vi "Untitled 5.vi"() -> ()   [LabVIEW 2023]
panel:
  in  "index":i8
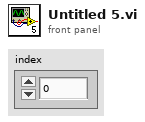
[diagram p1: front panel]
types:
  T1 = enum16{"plate1", "plate2", "plate3", "rinse", "seat"}
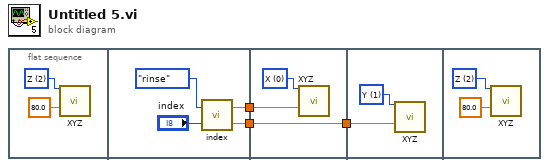
[diagram p0: block diagram]
diagram:
  n1 = flat-sequence {
    tunnel: [w9] -> w3
    tunnel: [w8] -> w1
    tunnel: w3 -> [w12]
    tunnel: [w10] -> w2
    tunnel: w1 -> [w10]
    tunnel: w2 -> [w13]
    frame #0 {
      w5 = u16 2 items=["X", "Y", "Z"] ("AXIS")
      n2 = call "XYZ.vi"("AXIS"=w5, "Set location (mm)"=80.0) -> ()  [unwired: 9 in, 5 out]
    }
    frame #1 {
      n3 = call "index.vi"("index"="index", "where"=T1."rinse") -> ("Y"=w8:dbl, "X"=w9:dbl)
    }
    frame #2 {
      w11 = u16 0 items=["X", "Y", "Z"] ("AXIS")
      n4 = call "XYZ.vi"("AXIS"=w11, "Set location (mm)"=w12) -> ()  [unwired: 9 in, 5 out]
    }
    frame #3 {
      w14 = u16 1 items=["X", "Y", "Z"] ("AXIS")
      n5 = call "XYZ.vi"("AXIS"=w14, "Set location (mm)"=w13) -> ()  [unwired: 9 in, 5 out]
    }
    frame #4 {
      w16 = u16 2 items=["X", "Y", "Z"] ("AXIS")
      n6 = call "XYZ.vi"("AXIS"=w16, "Set location (mm)"=80.0) -> ()  [unwired: 9 in, 5 out]
    }
  }
